vi "Library Collect VI Control Refnums.vi"(0 "VI refnum in":refnum<vi>, 11 "error in (no error)":errorcluster) -> (4 "VI refnum out":refnum<vi>, 8 "control refnums":refnum<vi>[](array[refnum]), 15 "error out":errorcluster)   [LabVIEW 2012]
doc: "Collect control refnums of a VI's panel. It recursively collects controls contained directly in the panel, as well as controls contained in the pages of a tab control, etc. Once done with the refnums, they must be closed in order to release the associated memory, at least for LabVIEW <= 7."
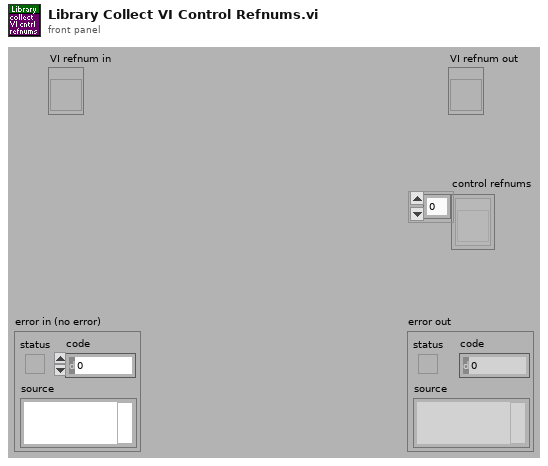
[diagram p1: front panel]
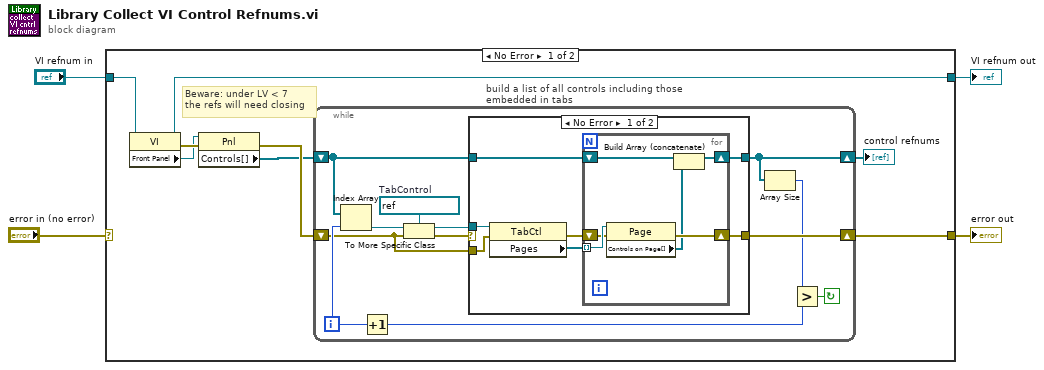
[diagram p0: block diagram]
diagram:
  n1 = case shown="No Error" "error in (no error)" {
    selector: "error in (no error)" -> [_ w41]
    tunnel: [w7 w41] -> w4
    tunnel: "VI refnum in" -> [w6 w40]
    tunnel: [w5 w40] -> w1
    frame No Error {
      # "Beware: under LV < 7\nthe refs will need closing"
      n2 = property class="VI"(reference=w6) -> (reference out=w5:refnum<vi>, error out=w10:errorcluster, "Front Panel"=w9:refnum<vi>)  [unwired: 1 in]
      n3 = property class="Pnl"(reference=w9, error in=w10) -> (error out=w12:errorcluster, "Controls[]"=w11:refnum<vi>[])  [unwired: 1 out]
      n4 = while "build a list of all controls including those embedded in tabs" {
        shift-left: w12 -> [w13]
        shift-right: [w20] -> w7
        shift-left: w11 -> [w23]
        shift-right: [w19] -> w8
        i -> [w24]
        stop <- w21 continue-if-true
        w17 = refnum<vi> refnum  # TabControl
        n5 = Index Array(array=w23, index=w24) -> (element=w16:refnum<vi>)
        n6 = Increment(x=w24) -> (x+1=w22:i32)
        n7 = To More Specific Class(target class=w17, reference=w16, error in=w13) -> (specific class reference=w15:refnum<vi>, error out=w14:errorcluster)
        n8 = case shown="No Error" w14 {
          tunnel: [w27 w39] -> w19
          tunnel: w23 -> [w29 w39]
          tunnel: w15 -> [w26 _]
          tunnel: [w28 w38] -> w20
          tunnel: w13 -> [w25 w38]
          frame No Error {
            n9 = property class="TabCtl"(reference=w26, error in=w25) -> (error out=w30:errorcluster, "Pages"=w31:refnum<vi>[])  [unwired: 1 out]
            n10 = for {
              tunnel: w31 -> [w37] mode=indexing
              shift-right: [w35] -> w28
              shift-left: w30 -> [w36]
              shift-right: [w32] -> w27
              shift-left: w29 -> [w34]
              n11 = property class="Page"(reference=w37, error in=w36) -> (error out=w35:errorcluster, "Controls on Page[]"=w33:refnum<vi>[])  [unwired: 1 out]
              n12 = Build Array (concatenate)(w34, w33) -> (w32:refnum<vi>[])
            }
          }
          frame Error {
          }
        }
        n13 = Array Size(array=w19) -> (size(s)=w18:i32)
        n14 = Greater?(x=w18, y=w22) -> (0:w21:bool)
      }
      "control refnums" <- w8
    }
    frame Error {
    }
  }
  "error out" <- w4
  "VI refnum out" <- w1
